vi "Read Hydrogen Oil Temperature.vi"(0 "Session Handle in":T1, 11 "error in (no error)":errorcluster) -> (4 "Session Handle out":T1, 6 "H2 Temp":dbl, 8 "Seconds Updated":dbl, 15 "error out":errorcluster)   [LabVIEW 2015, in "Gas.lvclass"]
uses:
  Gas.lvclass
  Typedefs/Session Handle.ctl
panel:
  out "Success?":bool
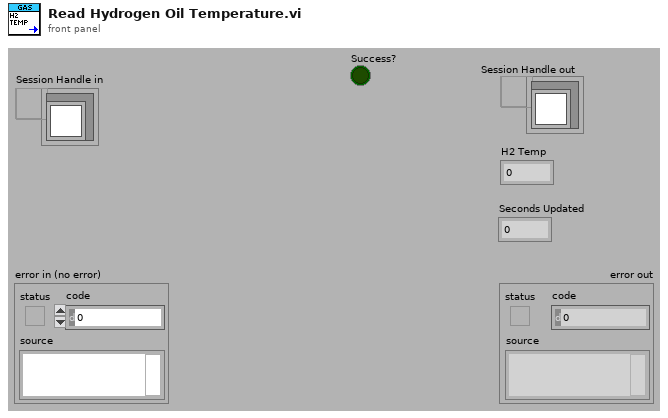
[diagram p1: front panel]
types:
  T1 = typedef "Gas.lvclass/Session Handle.ctl" = refnum<data-value>
  T2 = typedef "XNET Frame CAN.ctl" = cluster{"timestamp":timestamp, "payload":u8[], "identifier":u32, "type":T3, "extended?":bool, "echo?":bool}
  T3 = typedef "XNET Frame Type CAN.ctl" = u8
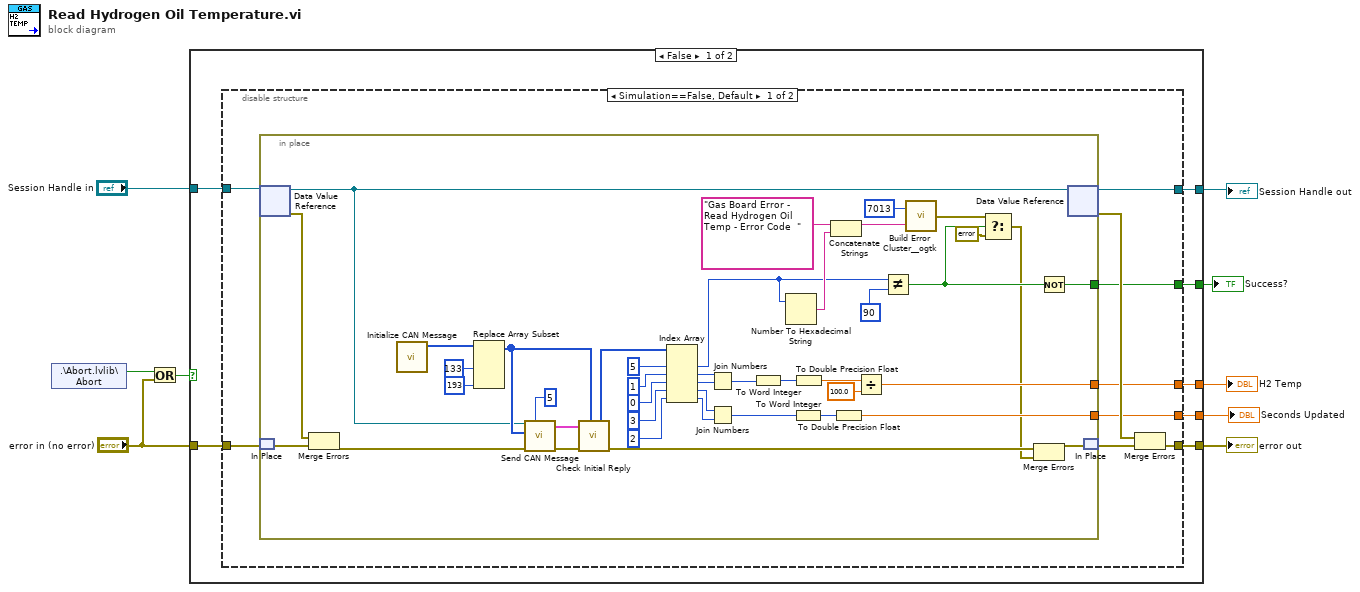
[diagram p0: block diagram]
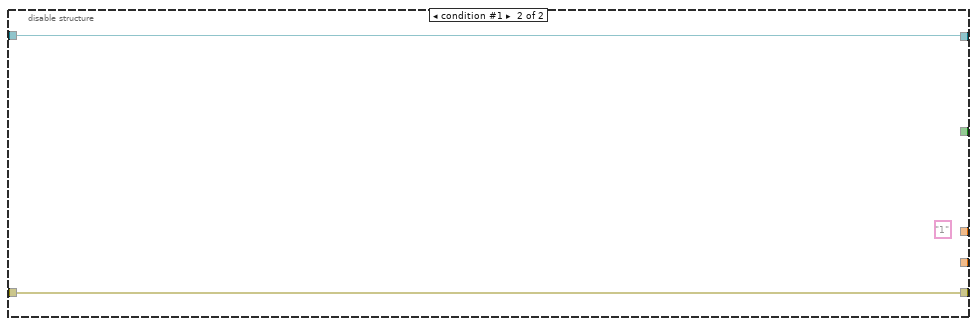
[diagram p2: hidden frame]
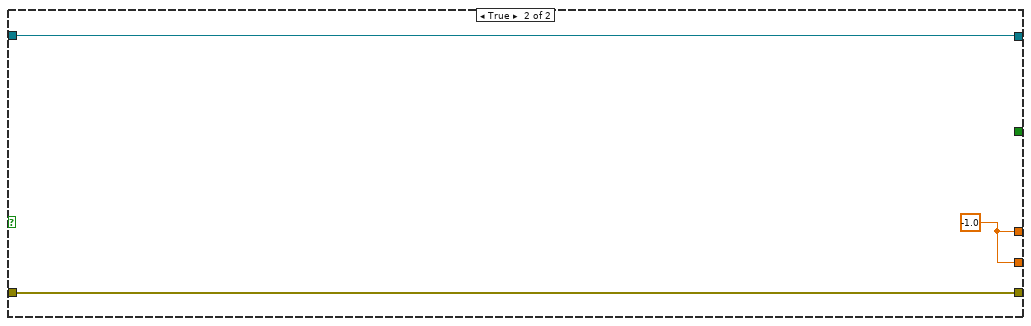
[diagram p3: hidden frame]
diagram:
  n1 = shared-variable ".\\Abort.lvlib\\Abort"() -> (w6:bool)  [unwired: 1 in, 1 out]
  n2 = Or(x=w6, y="error in (no error)") -> (x .or. y?=w4:bool)
  n3 = case shown="False" w4 {
    tunnel: [w16 w72] -> w8
    tunnel: [w15 w71] -> w7
    tunnel: "Session Handle in" -> [w14 w72]
    tunnel: "error in (no error)" -> [w13 w71]
    tunnel: [w12 w70] -> w3
    tunnel: [w11 w70] -> w2
    tunnel: [w10 _] -> w1
    frame False {
      n4 = disable-structure shown="Simulation==False, Default" {
        disable-tunnel: [w25 w69] -> w16
        disable-tunnel: [w22 w68] -> w15
        disable-tunnel: w14 -> [w21 w69]
        disable-tunnel: w13 -> [w20 w68]
        disable-tunnel: [w19 _] -> w12
        disable-tunnel: [w18 _] -> w11
        disable-tunnel: [w17 _] -> w10
        frame condition #0 (active) {
          n5 = in-place {
            in-place-border: [w35] -> w19
            in-place-border: [w32] -> w18
            in-place-border: [w48] -> w17
            n6 = in-place-dvr #1(w21) -> (w57:refnum<class "Gas.lvclass">, w62:errorcluster)
            n7 = in-place-match #2(w20) -> (w61:errorcluster)
            n8 = Merge Errors(w62, w61) -> (w56:errorcluster)
            n9 = call "Initialize CAN Message.vi"() -> ("Initial Payload"=w64:u8[])  [unwired: 11 in]
            n10 = Replace Array Subset(array=w64, new element #1=u8 133 ("new element/subarray"), new element #2=u8 193 ("new element/subarray")) -> (w60:u8[])  [unwired: 2 in]
            n11 = call "Send CAN Message.vi"("Number of Retries"=5, "error in (no error)"=w56, "payload"=w60, "Gas In"=w57) -> ("error out"=w28:errorcluster, "Reply"=w58:T2[])  [unwired: 5 in, 1 out]
            n12 = call "Check Initial Reply.vi"("Write Message"=w60, "error in (no error)"=w28, "Reply"=w58) -> ("error out"=w27:errorcluster, "Data Packet"=w63:u8[])  [unwired: 5 in, 2 out]
            n13 = Index Array(array=w63, index #1=5 ("index"), index #2=1 ("index"), index #3=0 ("index"), index #4=3 ("index"), index #5=2 ("index")) -> (element #1=w49:u8, element #2=w40:u8, element #3=w39:u8, element #4=w34:u8, element #5=w33:u8)
            n14 = Join Numbers(hi=w40, lo=w39) -> ((hi.lo)=w38:u16)
            n15 = Join Numbers(hi=w34, lo=w33) -> ((hi.lo)=w43:u16)
            n16 = To Word Integer(number=w38) -> (16bit integer=w41:i16)
            n17 = Number To Hexadecimal String(2:w49) -> (0:w53:string)  [unwired: 1 in]
            n18 = To Word Integer(number=w43) -> (16bit integer=w42:i16)
            n19 = To Double Precision Float(number=w41) -> (double precision float=w37:dbl)
            n20 = Concatenate Strings("Gas Board Error -  Read Hydrogen Oil Temp - Error Code  " ("string"), w53) -> (w52:string)
            n21 = To Double Precision Float(number=w42) -> (double precision float=w32:dbl)
            n22 = Divide(x=w37, y=100.0) -> (x/y=w35:dbl)
            n23 = Not Equal?(x=w49, y=u8 90 ("new element/subarray")) -> (x != y?=w29:bool)
            n24 = call <userlib>:"Build Error Cluster__ogtk.vi"("String to Prepend to source (\"\")"=w52, "code"=7013) -> ("error out"=w31:errorcluster)
            n25 = Select(t=w31, s=w29, f=errorcluster {"status"=FALSE, "code"=0, "source"=""}) -> (s? t:f=w26:errorcluster)
            n26 = Merge Errors(w27, w26) -> (w65:errorcluster)
            n27 = Not(x=w29) -> (.not. x?=w48:bool)
            n28 = in-place-dvr #1(w57) -> (w25:T1, w23:errorcluster)
            n29 = in-place-match #2(w65) -> (w24:errorcluster)
          }
          n30 = Merge Errors(w23, w24) -> (w22:errorcluster)
        }
        frame condition #1 {
          (unwired) "1"
        }
      }
    }
    frame True {
      w70 = -1.0
    }
  }
  "Session Handle out" <- w8
  "error out" <- w7
  "H2 Temp" <- w3
  "Seconds Updated" <- w2
  "Success?" <- w1
